vi "Get JSONEditor Events.vi"(8 "Error In":errorcluster, 11 "Component.JSONEditor in":refnum<class "Component.JSONEditor.lvclass">) -> (0 "Error Out":errorcluster, 2 "Events":T1, 3 "Component.JSONEditor out":refnum<class "Component.JSONEditor.lvclass">)   [LabVIEW 2020, in "Component.JSONEditor.lvclass"]
uses:
  Component.JSONEditor.lvclass
  private/JSONEditor Events.ctl
  private/JSON Updated Event Data--cluster.ctl
  private/Seleced Node Path Event Data--string.ctl
  Component.JSONEditor.lvclass/Component.JSONEditor.ctl
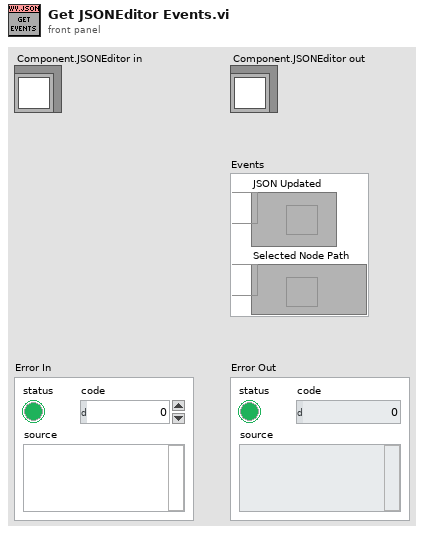
[diagram p1: front panel]
types:
  T1 = typedef "Component.JSONEditor.lvclass/JSONEditor Events.ctl" = cluster{"JSON Updated":refnum<user-event>, "Selected Node Path":refnum<user-event>}
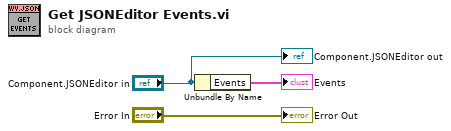
[diagram p0: block diagram]
diagram:
  n1 = Unbundle By Name("Component.JSONEditor in") -> ("Events"=→"Events":T1)
  "Error Out" <- "Error In"
  "Component.JSONEditor out" <- "Component.JSONEditor in"
